vi "CODMn启动命令.vi"(11 "参数":T1={"站号"=21, "量程切换"=enum."AUTO", "控制命令"=0, "模式设置"=enum."待机", "测量间隔"=0} {"站号" items=["CODMn"=21, "总氮"=2, "氨氮"=3]; "控制命令" items=["启动测量"=1, "标样核查"=2, "零点核查"=3, "跨度核查"=4, "空白测试"=5, "平行样测试"=6, "加标回收"=7, "空白校准"=8, "标样校准"=9, "初始化（清洗）"=10, "停止测试"=11, "仪器重启"=12, "校时"=13, "模式设置"=14, "测量间隔设置"=15, "调试"=22, "填充管路"=30, "清洗管路"=31, "清洗反应杯"=32]}) -> (3 "启动命令":cluster{"命令":string, "data":variant})   [LabVIEW 2016, in "斯坦道CODMn新电路板.lvlib"]
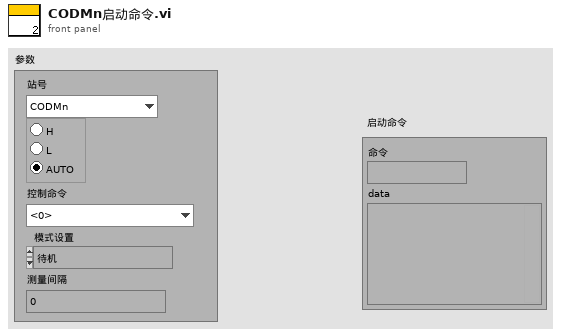
[diagram p1: front panel]
types:
  T1 = cluster{"站号":u16, "量程切换":enum32{"H", "L", "AUTO"}, "控制命令":u16, "模式设置":enum16{"待机", "连续模式", "周期模式", "定点模式", "受控模式", "手动模式"}, "测量间隔":u16}
  T2 = enum16{"待机", "连续模式", "周期模式", "定点模式", "受控模式", "手动模式"}
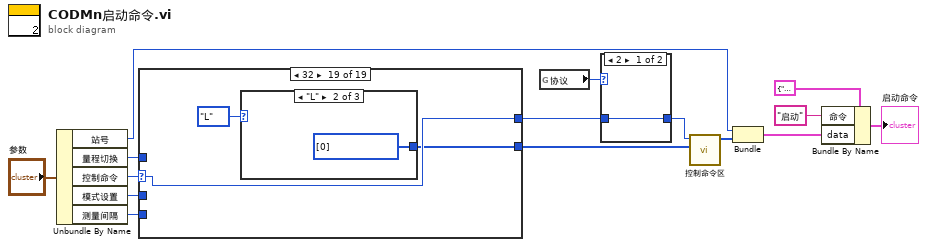
[diagram p0: block diagram]
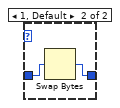
[diagram p2: hidden frame]
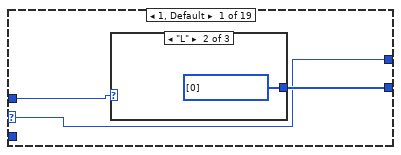
[diagram p3: hidden frame]
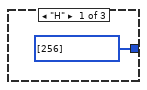
[diagram p4: hidden frame]
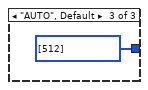
[diagram p5: hidden frame]
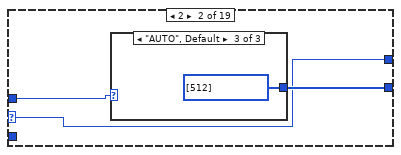
[diagram p6: hidden frame]
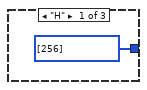
[diagram p7: hidden frame]
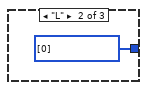
[diagram p8: hidden frame]
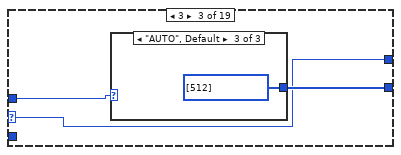
[diagram p9: hidden frame]
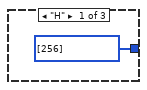
[diagram p10: hidden frame]
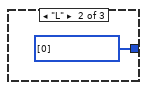
[diagram p11: hidden frame]
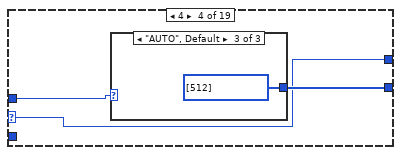
[diagram p12: hidden frame]
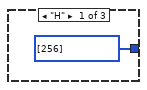
[diagram p13: hidden frame]
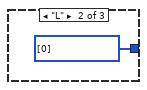
[diagram p14: hidden frame]
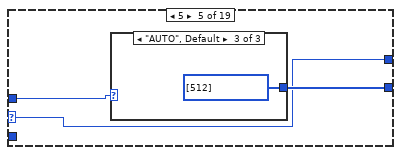
[diagram p15: hidden frame]
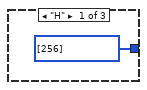
[diagram p16: hidden frame]
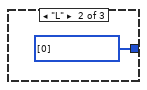
[diagram p17: hidden frame]
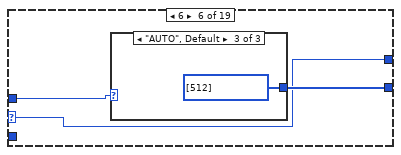
[diagram p18: hidden frame]
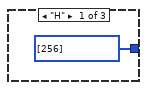
[diagram p19: hidden frame]
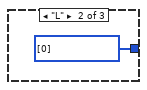
[diagram p20: hidden frame]
diagram:
  n1 = Unbundle By Name("参数") -> ("站号"=w13:u16, "量程切换"=w12:enum32{"H", "L", "AUTO"}, "控制命令"=w11:u16, "模式设置"=w9:T2, "测量间隔"=w10:u16)
  n2 = case shown="32" w11 {
    selector: w11 -> [w16 w22 w28 w34 w40 w46 w52 w58 w64 w70 w72 w74 w76 w81 w91 w98 w104 w110 w116]
    tunnel: [w18 w24 w29 w35 w41 w48 w54 w60 w66 i32[] [] i32[] [] i32[] [] w77 w83 w93 w97 w103 w109 w115] -> w4
    tunnel: w12 -> [w17 w23 w30 w36 w42 w47 w53 w59 w65 _ _ _ _ _ _ w96 _ _ _]
    tunnel: [w16 w22 w28 w34 w40 w46 w52 w58 w64 w70 w72 w74 w76 w81 w91 w98 w104 w110 w116] -> w3
    tunnel: w10 -> [_ _ _ _ _ _ _ _ _ _ _ _ _ _ w92 _ _ _ _]
    tunnel: w9 -> [_ _ _ _ _ _ _ _ _ _ _ _ _ w82 _ _ _ _ _]
    frame 1, Default {
      n3 = case shown="\"L\"" w17 {
        tunnel: [i32[] [256] i32[] [0] i32[] [512]] -> w18
        frame "H" {
        }
        frame "L" {
        }
        frame "AUTO", Default {
        }
      }
    }
    frame 2 {
      n4 = case shown="\"AUTO\", Default" w23 {
        tunnel: [i32[] [256] i32[] [0] i32[] [512]] -> w24
        frame "H" {
        }
        frame "L" {
        }
        frame "AUTO", Default {
        }
      }
    }
    frame 3 {
      n5 = case shown="\"AUTO\", Default" w30 {
        tunnel: [i32[] [256] i32[] [0] i32[] [512]] -> w29
        frame "H" {
        }
        frame "L" {
        }
        frame "AUTO", Default {
        }
      }
    }
    frame 4 {
      n6 = case shown="\"AUTO\", Default" w36 {
        tunnel: [i32[] [256] i32[] [0] i32[] [512]] -> w35
        frame "H" {
        }
        frame "L" {
        }
        frame "AUTO", Default {
        }
      }
    }
    frame 5 {
      n7 = case shown="\"AUTO\", Default" w42 {
        tunnel: [i32[] [256] i32[] [0] i32[] [512]] -> w41
        frame "H" {
        }
        frame "L" {
        }
        frame "AUTO", Default {
        }
      }
    }
    frame 6 {
      n8 = case shown="\"AUTO\", Default" w47 {
        tunnel: [i32[] [256] i32[] [0] i32[] [512]] -> w48
        frame "H" {
        }
        frame "L" {
        }
        frame "AUTO", Default {
        }
      }
    }
    frame 7 {
      n9 = case shown="\"AUTO\", Default" w53 {
        tunnel: [i32[] [256] i32[] [0] i32[] [512]] -> w54
        frame "H" {
        }
        frame "L" {
        }
        frame "AUTO", Default {
        }
      }
    }
    frame 8 {
      n10 = case shown="\"AUTO\", Default" w59 {
        tunnel: [i32[] [256] i32[] [0] i32[] [512]] -> w60
        frame "H" {
        }
        frame "L" {
        }
        frame "AUTO", Default {
        }
      }
    }
    frame 9 {
      n11 = case shown="\"AUTO\", Default" w65 {
        tunnel: [i32[] [256] i32[] [0] i32[] [512]] -> w66
        frame "H" {
        }
        frame "L" {
        }
        frame "AUTO", Default {
        }
      }
    }
    frame 10 {
    }
    frame 11 {
    }
    frame 12 {
    }
    frame 13 {
      n12 = Get Date/Time In Seconds() -> (seconds since 1Jan1904=w80:timestamp)
      n13 = Insert Into Array(array=timestamp[] [] ("数组"), new element=w80) -> (w78:timestamp[])  [unwired: 1 in]
      n14 = call "DateToHex.vi"("DATE"=w78) -> ("数组"=w77:u16[])  [unwired: 10 in]
    }
    frame 14 {
      n15 = case shown="\"定点模式\"" w82 {
        tunnel: [i32[] [0] i32[] [1] i32[] [2] i32[] [3] i32[] [4] i32[] [5]] -> w84
        frame "待机", Default {
        }
        frame "连续模式" {
        }
        frame "周期模式" {
        }
        frame "定点模式" {
        }
        frame "受控模式" {
        }
        frame "手动模式" {
        }
      }
      n16 = call "HexToWord.vi"("数组"=w84) -> ("WORD"=w83:u16[])  [unwired: 10 in]
    }
    frame 15 {
      n17 = Replace Array Subset(array=i32[] [0], new element=w92) -> (w94:i32[])  [unwired: 1 in]
      n18 = call "HexToWord.vi"("数组"=w94) -> ("WORD"=w93:u16[])  [unwired: 10 in]
    }
    frame 22 {
      n19 = case shown="\"L\"" w96 {
        tunnel: [i32[] [256] i32[] [0] i32[] [512]] -> w97
        frame "H" {
        }
        frame "L" {
        }
        frame "AUTO", Default {
        }
      }
    }
    frame 30 {
      n20 = case shown="\"L\"" enum32{"H", "L", "AUTO"}."L" ("量程切换") {
        tunnel: [i32[] [256] i32[] [0] i32[] [512]] -> w103
        frame "H" {
        }
        frame "L" {
        }
        frame "AUTO", Default {
        }
      }
    }
    frame 31 {
      n21 = case shown="\"L\"" enum32{"H", "L", "AUTO"}."L" ("量程切换") {
        tunnel: [i32[] [256] i32[] [0] i32[] [512]] -> w109
        frame "H" {
        }
        frame "L" {
        }
        frame "AUTO", Default {
        }
      }
    }
    frame 32 {
      n22 = case shown="\"L\"" enum32{"H", "L", "AUTO"}."L" ("量程切换") {
        tunnel: [i32[] [256] i32[] [0] i32[] [512]] -> w115
        frame "H" {
        }
        frame "L" {
        }
        frame "AUTO", Default {
        }
      }
    }
  }
  n23 = global read "CODMn断电保存全局变量.vi" "协议"() -> (w1:u16)
  n24 = case shown="2" w1 {
    tunnel: w3 -> [w120 w122]
    tunnel: [w120 w121] -> w2
    frame 2 {
    }
    frame 1, Default {
      n25 = Swap Bytes(anything=w122) -> (byte swapped=w121:u16)
    }
  }
  n26 = call "控制命令区.vi"("控制命令参数"=w4, "控制命令"=w2) -> ("控制命令"=w8:u16[])  [unwired: 9 in]
  n27 = Bundle("站号"=w13, "控制命令"=w8) -> (w5:cluster{"站号":u16, "控制命令":u16[]})  [unwired: 1 in]
  n28 = Bundle By Name(cluster=cluster{"命令":string, "data":variant} {"命令"="", "data"=variant} ("元素"), "命令"="启动", "data"=w5) -> (→"启动命令":cluster{"命令":string, "data":variant})
